vi "Get settings path.vi"(8 "error in (no error)":errorcluster, 11 "Autofocus in":refnum<class "Autofocus.lvclass">) -> (0 "error out":errorcluster, 2 "settings path":path, 3 "Autofocus out":refnum<class "Autofocus.lvclass">)   [LabVIEW 2012, in "Autofocus.lvclass"]
doc: "Returns the settings path."
uses:
  Autofocus.lvclass
  <vilib>/Distrio/Murmex/Murmex/Murmex.lvclass
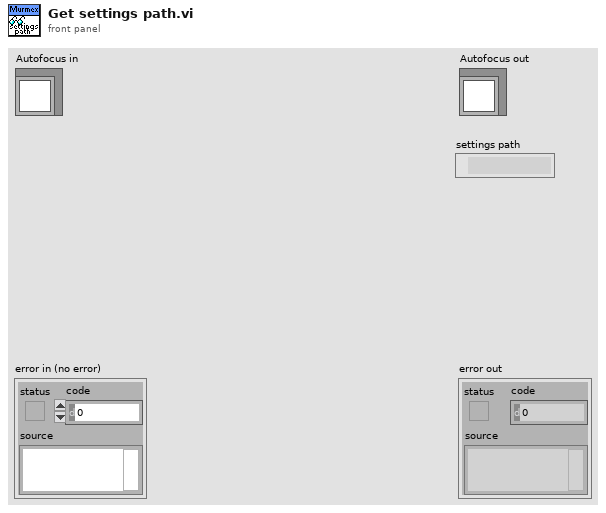
[diagram p1: front panel]
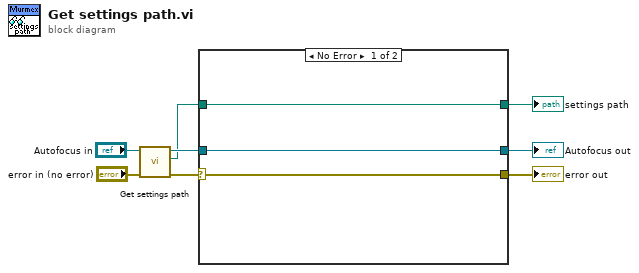
[diagram p0: block diagram]
diagram:
  n1 = call-parent "Get settings path.vi"("error in (no error)"="error in (no error)", "Murmex in"="Autofocus in") -> ("error out"=w6:errorcluster, "settings path"=w2:path, "Murmex out"=w5:refnum<class "Autofocus.lvclass">)  [unwired: 7 in]
  n2 = case shown="No Error" w6 {
    selector: w6 -> [w11 w14]
    tunnel: w5 -> [w10 w13]
    tunnel: [w11 w14] -> w4
    tunnel: [w10 w13] -> w3
    tunnel: w2 -> [w9 w12]
    tunnel: [w9 w12] -> w1
    frame No Error {
    }
    frame Error {
    }
  }
  "error out" <- w4
  "Autofocus out" <- w3
  "settings path" <- w1
